vi "Remove 2D Array Global Outliers (U16) with Mask.vi"(6 "Init?":bool, 8 "Error In":errorcluster, 9 "2D Mask in":bool[][](array[boolean]), 11 "2D Array in":u16[][](array[numeric])) -> (0 "Error Out":errorcluster, 1 "Hot Pixel Locations":cluster{"Numeric":i32, "Numeric":i32}[](array[cluster]), 2 "# Modified Values":i32, 3 "2D Array out":u16[][](array[numeric]))   [LabVIEW 2021]
uses:
  <vilib>/Utility/error.llb/Error Cluster From Error Code.vi
  <vilib>/ErrorRing/Error Ring.xnode
panel:
  out "CPU (s)":dbl
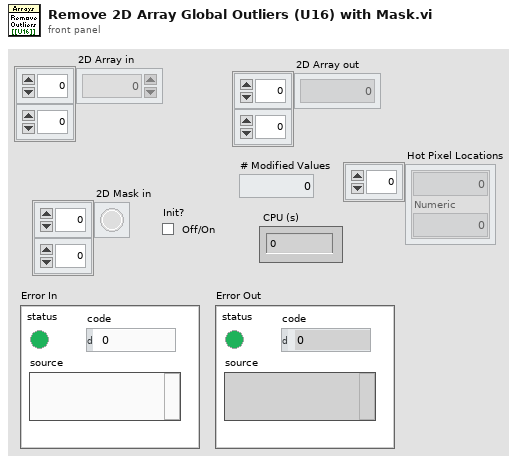
[diagram p1: front panel]
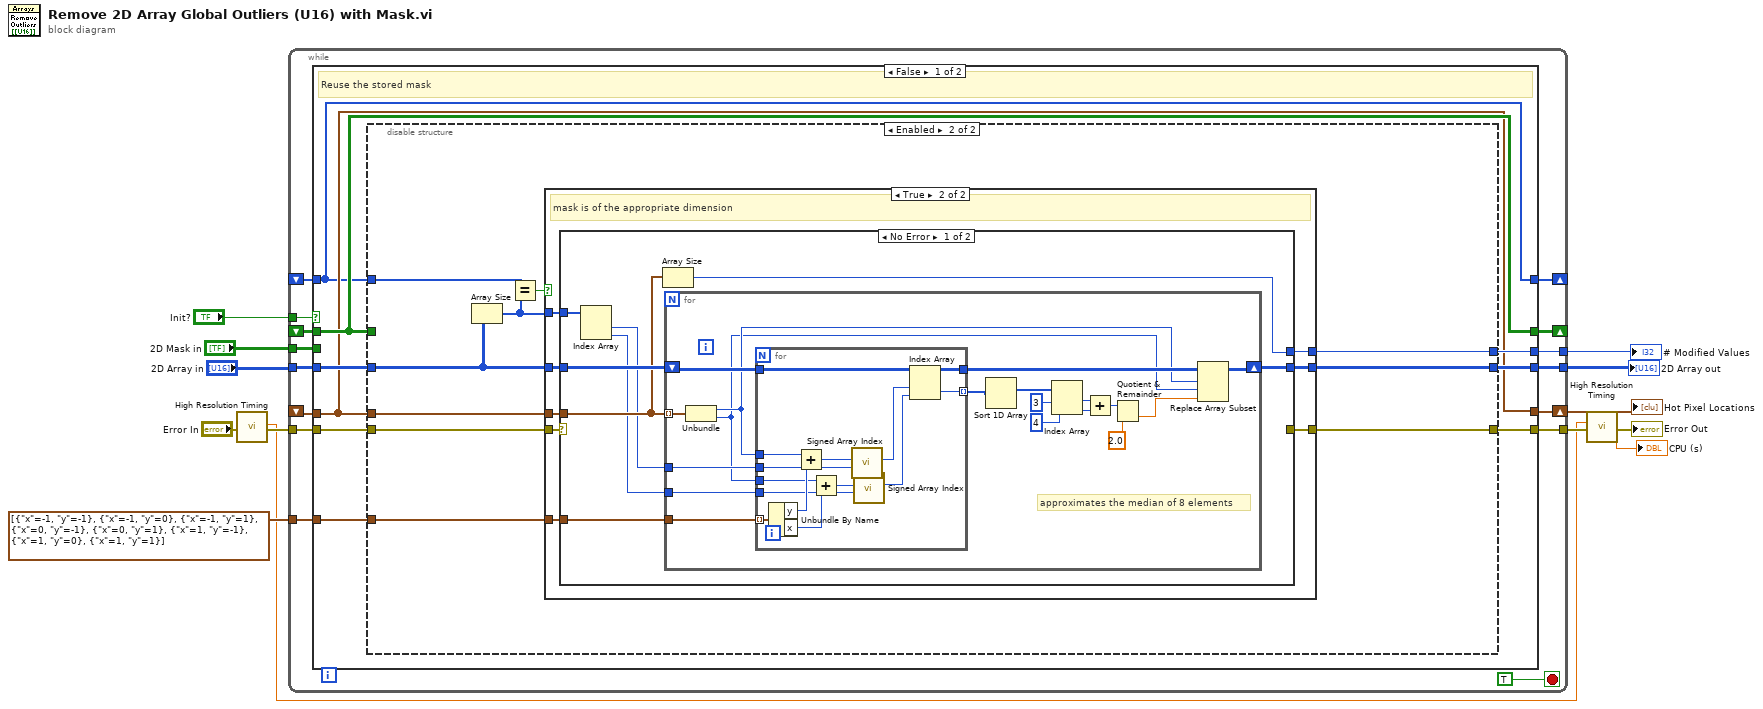
[diagram p0: block diagram]
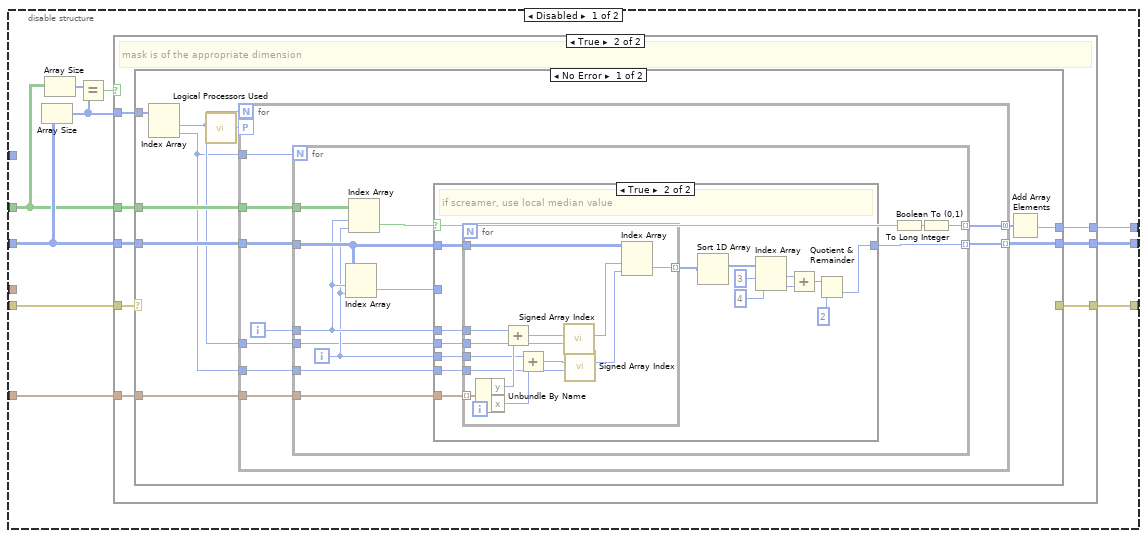
[diagram p2: hidden frame]
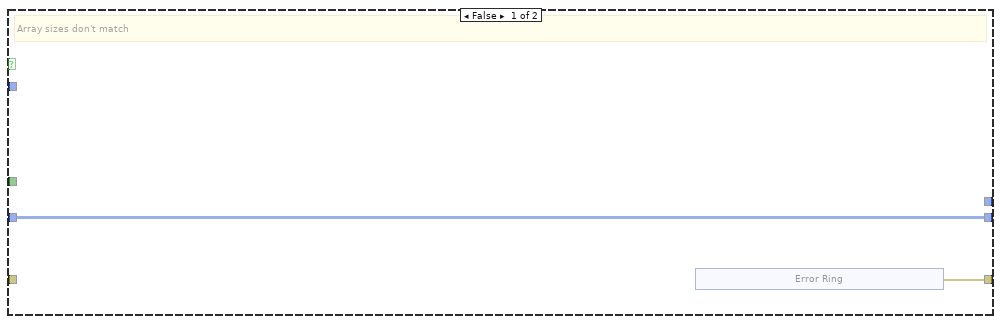
[diagram p3: hidden frame]
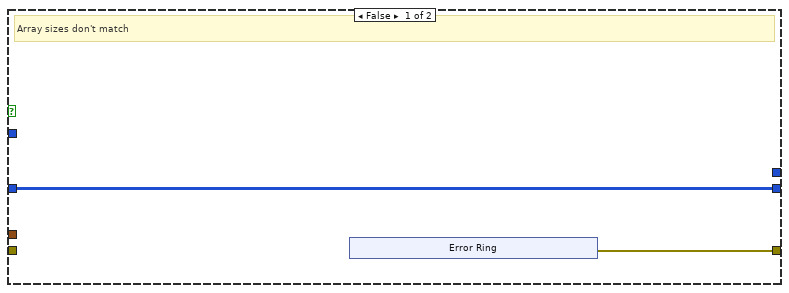
[diagram p6: hidden frame]
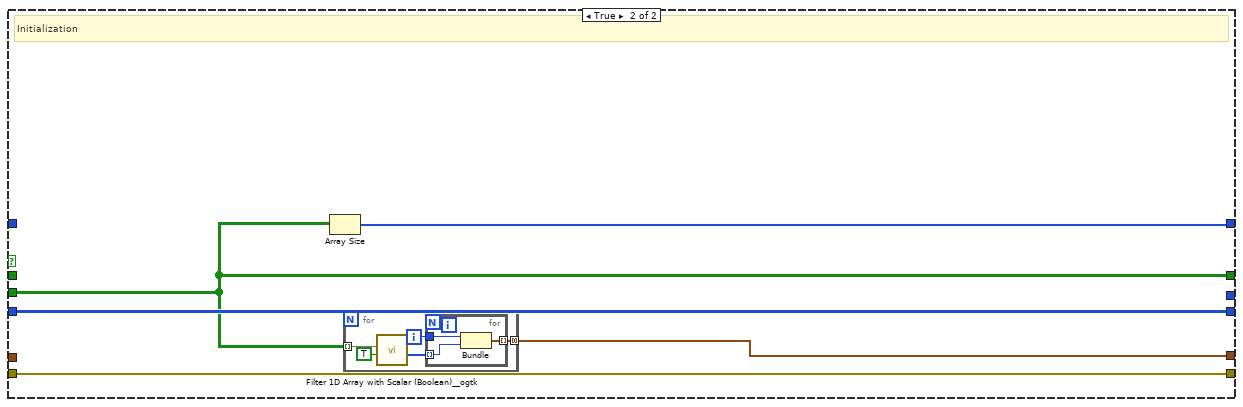
[diagram p8: hidden frame]
diagram:
  n1 = call "High Resolution Timing.vi"("Error In"="Error In") -> ("elapsed (relative) seconds"=w3:dbl, "Error Out"=w5:errorcluster)  [unwired: 16 in, 1 out]
  n2 = while {
    tunnel: cluster{"x":i32, "y":i32}[] [{"x"=-1, "y"=-1}, {"x"=-1, "y"=0}, {"x"=-1, "y"=1}, {"x"=0, "y"=-1}, {"x"=0, "y"=1}, {"x"=1, "y"=-1}, {"x"=1, "y"=0}, {"x"=1, "y"=1}] -> [w27]
    tunnel: [w23] -> w8
    tunnel: "Init?" -> [w22]
    tunnel: "2D Array in" -> [w28]
    tunnel: [w24] -> w9
    shift-right: [w20] -> _
    shift-left: _ -> [w18]
    tunnel: "2D Mask in" -> [w19]
    tunnel: w5 -> [w26]
    tunnel: [w25] -> w10
    shift-right: [w17] -> w1
    shift-left: _ -> [w15]
    shift-right: [w16] -> _
    shift-left: _ -> [w14]
    stop <- TRUE stop-if-true
    n3 = case shown="False" w22 {
      tunnel: w28 -> [w37 w192]
      tunnel: w27 -> [w36 _]
      tunnel: w26 -> [w35 w193]
      tunnel: [w34 w193] -> w25
      tunnel: [w33 w192] -> w24
      tunnel: [w32 _] -> w23
      tunnel: [w31 w191] -> w20
      tunnel: w19 -> [_ w191]
      tunnel: w18 -> [w31 _]
      tunnel: [w30 w190] -> w17
      tunnel: [w29 w189] -> w16
      tunnel: w15 -> [w30 _]
      tunnel: w14 -> [w29 _]
      frame False {
        # "Reuse the stored mask"
        n4 = disable-structure shown="Enabled" {
          disable-tunnel: w37 -> [w47 w128]
          disable-tunnel: w36 -> [w46 w131]
          disable-tunnel: w35 -> [w45 w130]
          disable-tunnel: [w44 w129] -> w34
          disable-tunnel: [w43 w127] -> w33
          disable-tunnel: [w42 w126] -> w32
          disable-tunnel: w31 -> [w38 _]
          disable-tunnel: w30 -> [_ w125]
          disable-tunnel: w29 -> [_ w124]
          frame Disabled {
            n5 = Array Size(array=w47) -> (size(s)=w40:i32[])
            n6 = Array Size(array=w38) -> (size(s)=w41:i32[])
            n7 = Equal?(x=w41, y=w40) -> (x = y?=w39:bool)
            n8 = case shown="True" w39 {
              tunnel: w47 -> [w49 w61]
              tunnel: w46 -> [_ w60]
              tunnel: w45 -> [_ w59]
              tunnel: [w48 w58] -> w44
              tunnel: [w49 w57] -> w43
              tunnel: [_ w56] -> w42
              tunnel: w40 -> [_ w55]
              tunnel: w38 -> [_ w54]
              frame False {
                # "Array sizes don't match"
                n9 = xnode "Error Ring"() -> ("error out"=w48:errorcluster)
              }
              frame True {
                # "mask is of the appropriate dimension"
                n10 = case shown="No Error" w59 {
                  selector: w59 -> [_ w122]
                  tunnel: w60 -> [w71 _]
                  tunnel: [w70 w123] -> w57
                  tunnel: w61 -> [w69 w123]
                  tunnel: w55 -> [w68 _]
                  tunnel: [_ w122] -> w58
                  tunnel: [w64 _] -> w56
                  tunnel: w54 -> [w65 _]
                  frame No Error {
                    n11 = Index Array(array=w68) -> (element #1=w63:i32, element #2=w62:i32)  [unwired: 2 in]
                    n12 = call "Logical Processors Used.vi"() -> ("# Logical Processor Used"=w67:i32)  [unwired: 6 in]
                    n13 = for {
                      N: w63 -> [_]
                      tunnel: w69 -> [w80]
                      tunnel: w71 -> [w79]
                      tunnel: [w78] -> w70 mode=indexing
                      tunnel: w62 -> [w77]
                      workers-P: w67 -> [_]
                      tunnel: [w75] -> w66 mode=concatenating
                      tunnel: w65 -> [w74]
                      tunnel: w63 -> [w73]
                      tunnel: w62 -> [w72]
                      i -> [w76]
                      n14 = for {
                        N: w77 -> [_]
                        tunnel: w76 -> [w90]
                        tunnel: w80 -> [w91]
                        tunnel: w79 -> [w92]
                        tunnel: [w89] -> w78 mode=indexing
                        tunnel: [w85] -> w75 mode=indexing
                        tunnel: w74 -> [w84]
                        tunnel: w73 -> [w82]
                        tunnel: w72 -> [w81]
                        i -> [w88]
                        n15 = Index Array(array=w91, index (row)=w90, index (col)=w88) -> (element=w83:u16)
                        n16 = Index Array(array=w84, index (row)=w90, index (col)=w88) -> (element=w87:bool)
                        n17 = case shown="True" w87 {
                          tunnel: w92 -> [_ w108]
                          tunnel: w91 -> [_ w101]
                          tunnel: w90 -> [_ w100]
                          tunnel: w88 -> [_ w99]
                          tunnel: [w93 w98] -> w89
                          tunnel: w83 -> [w93 _]
                          tunnel: w82 -> [_ w95]
                          tunnel: w81 -> [_ w94]
                          frame False {
                            # "if value < percentile value, keep it"
                          }
                          frame True {
                            # "if screamer, use local median value"
                            n18 = for {
                              tunnel: w101 -> [w116]
                              tunnel: w108 -> [w121] mode=indexing
                              tunnel: w100 -> [w120]
                              tunnel: w99 -> [w118]
                              tunnel: [w115] -> w97 mode=indexing
                              tunnel: w95 -> [w112]
                              tunnel: w94 -> [w109]
                              n19 = Unbundle By Name(w121) -> ("y"=w119:i32, "x"=w117:i32)
                              n20 = Add(x=w120, y=w119) -> (x+y=w114:i32)
                              n21 = Add(x=w118, y=w117) -> (x+y=w111:i32)
                              n22 = call "Signed Array Index.vi"("Array Size"=w112, "Array Index in"=w114) -> ("Array Index out"=w113:i32)  [unwired: 9 in]
                              n23 = call "Signed Array Index.vi"("Array Size"=w109, "Array Index in"=w111) -> ("Array Index out"=w110:i32)  [unwired: 9 in]
                              n24 = Index Array(array=w116, index (row)=w113, index (col)=w110) -> (element=w115:u16)
                            }
                            n25 = Sort 1D Array(array=w97) -> (sorted array=w96:u16[])
                            n26 = Index Array(array=w96, index #1=3 ("index"), index #2=4 ("index")) -> (element #1=w105:u16, element #2=w104:u16)
                            n27 = Add(x=w105, y=w104) -> (x+y=w103:u16)
                            n28 = Quotient & Remainder(x=w103, y=u16 2) -> (floor(x/y)=w98:u16)  [unwired: 1 out]
                          }
                        }
                        n29 = Boolean To (0,1)(Boolean=w87) -> (0, 1=w86:i16)
                        n30 = To Long Integer(number=w86) -> (32bit integer=w85:i32)
                      }
                    }
                    n31 = Add Array Elements(numeric array=w66) -> (sum=w64:i32)
                  }
                  frame Error {
                  }
                }
              }
            }
          }
          frame Enabled {
            n32 = Array Size(array=w128) -> (size(s)=w133:i32[])
            n33 = Equal?(x=w124, y=w133) -> (x = y?=w132:bool)
            n34 = case shown="True" w132 {
              tunnel: w128 -> [w135 w147]
              tunnel: w131 -> [_ w146]
              tunnel: w130 -> [_ w145]
              tunnel: [w134 w144] -> w129
              tunnel: [w135 w143] -> w127
              tunnel: [_ w142] -> w126
              tunnel: w133 -> [_ w141]
              tunnel: w125 -> [_ w140]
              frame False {
                # "Array sizes don't match"
                n35 = xnode "Error Ring"() -> ("error out"=w134:errorcluster)
              }
              frame True {
                # "mask is of the appropriate dimension"
                n36 = case shown="No Error" w145 {
                  selector: w145 -> [_ w187]
                  tunnel: w146 -> [w155 _]
                  tunnel: [w150 w188] -> w143
                  tunnel: w147 -> [w154 w188]
                  tunnel: w141 -> [w153 _]
                  tunnel: [_ w187] -> w144
                  tunnel: [w151 _] -> w142
                  tunnel: w140 -> [w152 _]
                  frame No Error {
                    n37 = Index Array(array=w153) -> (element #1=w149:i32, element #2=w148:i32)  [unwired: 2 in]
                    n38 = Array Size(array=w152) -> (size(s)=w151:i32)
                    n39 = for {
                      tunnel: w155 -> [w172]
                      tunnel: w149 -> [w171]
                      tunnel: w148 -> [w170]
                      tunnel: w152 -> [w169] mode=indexing
                      shift-right: [w159] -> w150
                      shift-left: w154 -> [w173]
                      # "approximates the median of 8 elements"
                      n40 = Unbundle(w169) -> (w157:i32, "Numeric"=w156:i32)
                      n41 = for {
                        tunnel: w173 -> [w174]
                        tunnel: w172 -> [w186] mode=indexing
                        tunnel: w157 -> [w185]
                        tunnel: w156 -> [w183]
                        tunnel: [w181] -> w162 mode=indexing
                        tunnel: w171 -> [w178]
                        tunnel: w170 -> [w175]
                        tunnel: [w174] -> w160
                        n42 = Unbundle By Name(w186) -> ("y"=w184:i32, "x"=w182:i32)
                        n43 = Add(x=w185, y=w184) -> (x+y=w180:i32)
                        n44 = Add(x=w183, y=w182) -> (x+y=w177:i32)
                        n45 = call "Signed Array Index.vi"("Array Size"=w178, "Array Index in"=w180) -> ("Array Index out"=w179:i32)  [unwired: 9 in]
                        n46 = call "Signed Array Index.vi"("Array Size"=w175, "Array Index in"=w177) -> ("Array Index out"=w176:i32)  [unwired: 9 in]
                        n47 = Index Array(array=w174, index (row)=w179, index (col)=w176) -> (element=w181:u16)
                      }
                      n48 = Sort 1D Array(array=w162) -> (sorted array=w161:u16[])
                      n49 = Index Array(array=w161, index #1=3 ("index"), index #2=4 ("index")) -> (element #1=w166:u16, element #2=w165:u16)
                      n50 = Add(x=w166, y=w165) -> (x+y=w164:u16)
                      n51 = Quotient & Remainder(x=w164, y=sgl 2.0) -> (floor(x/y)=w158:sgl)  [unwired: 1 out]
                      n52 = Replace Array Subset(array=w160, new element=w158, index (row)=w157, index (col)=w156) -> (w159:u16[][])
                    }
                  }
                  frame Error {
                  }
                }
              }
            }
          }
        }
      }
      frame True {
        # "Initialization"
        n53 = Array Size(array=w191) -> (size(s)=w189:i32[])
        n54 = for {
          tunnel: w191 -> [w198] mode=indexing
          tunnel: [w194] -> w190 mode=concatenating
          i -> [w195]
          n55 = call <userlib>:"Filter 1D Array with Scalar (Boolean)__ogtk.vi"("items to filter"=TRUE ("Boolean"), "array"=w198) -> ("filtered item indices"=w196:i32[])  [unwired: 4 in, 1 out]
          n56 = for {
            tunnel: w196 -> [w200] mode=indexing
            tunnel: w195 -> [w201]
            tunnel: [w199] -> w194 mode=indexing
            n57 = Bundle(w201, "Numeric"=w200) -> (w199:cluster{i32, "Numeric":i32})  [unwired: 1 in]
          }
        }
      }
    }
  }
  "2D Array out" <- w9
  "# Modified Values" <- w8
  "Hot Pixel Locations" <- w1
  n58 = call "High Resolution Timing.vi"("relative seconds (NaN)"=w3, "Error In"=w10) -> ("elapsed (relative) seconds"=→"CPU (s)":dbl, "Error Out"=→"Error Out":errorcluster)  [unwired: 15 in, 1 out]
